vi "PE_DataAcquisition_Expire.vi"() -> ()   [LabVIEW 2016]
uses:
  SerialSupport/Serial - Settings.ctl
  SerialSupport/Serial - XON-XOFF Characters.ctl
  SerialSupport/Serial - ASCII Characters.ctl
  <vilib>/Instr/_visa.llb/VISA Configure Serial Port (Instr).vi
  database/database.lvlib
panel:
  out "当前指令 2":string
  in  "标记 2":dbl
  in  "TestId 2":string
  out "CtrlCmdMsg":string
  out "串口信息发送持久化":bool=TRUE
  out "串口信息发送":bool=TRUE
  out "UDP发送持久化":bool=TRUE
  out "TCP发送持久化":bool=TRUE
  out "串口接收持久化":bool=TRUE
  in  "串口发送按钮":bool
  in  "Serial output":string caption="字符串输出"
  in  "终止符":u8=10 format="%.0x"
  in  "终止符时结束写入？":bool=TRUE
  in  "VISA资源名称":refnum<visa-resource-name>="COM10"
  in  "XON/XOFF字符":T1={"XON"=enum."DC1", "XOFF"=enum."DC3"}
  in  "串口设置":T3={"波特率"=115200, "数据位"=8, "校验"=enum."None", "停止位"=10, "流控制"=0} {"流控制" items=["无"=0, "XON/XOFF"=1, "RTS/CTS"=2, "DTR/DSR"=4]; "停止位" items=["1.0"=10, "1.5"=15, "2.0"=20]; "数据位" min=5 max=8 step=1; "波特率" items=["75"=75, "110"=110, "134"=134, "150"=150, "300"=300, "600"=600, "1200"=1200, "1800"=1800, "2400"=2400, "4800"=4800, "7200"=7200, "9600"=9600, "14400"=14400, "19200"=19200, "28800"=28800, "38400"=38400, "56000"=56000, "57600"=57600, "115200"=115200, "128000"=128000, "230400"=230400]}
  in  "终止符时结束读取？":bool=TRUE
  in  "读取":bool=TRUE
  in  "串口停止":bool
  in  "串口发送命令":string="{\"cmd\":\"CT_ON\",\"id\":\"C_FR\",on:true}"
  out "串口信息":string
  in  "串口最大字节":u32=1000
  out "当前指令":string
  in  "错误输入 16":errorcluster caption="错误输入"
  in  "TestId":string
  in  "dataLabel":string
  in  "content":string
  in  "msgid":dbl
  # "用于说明数据来源等 如串口"
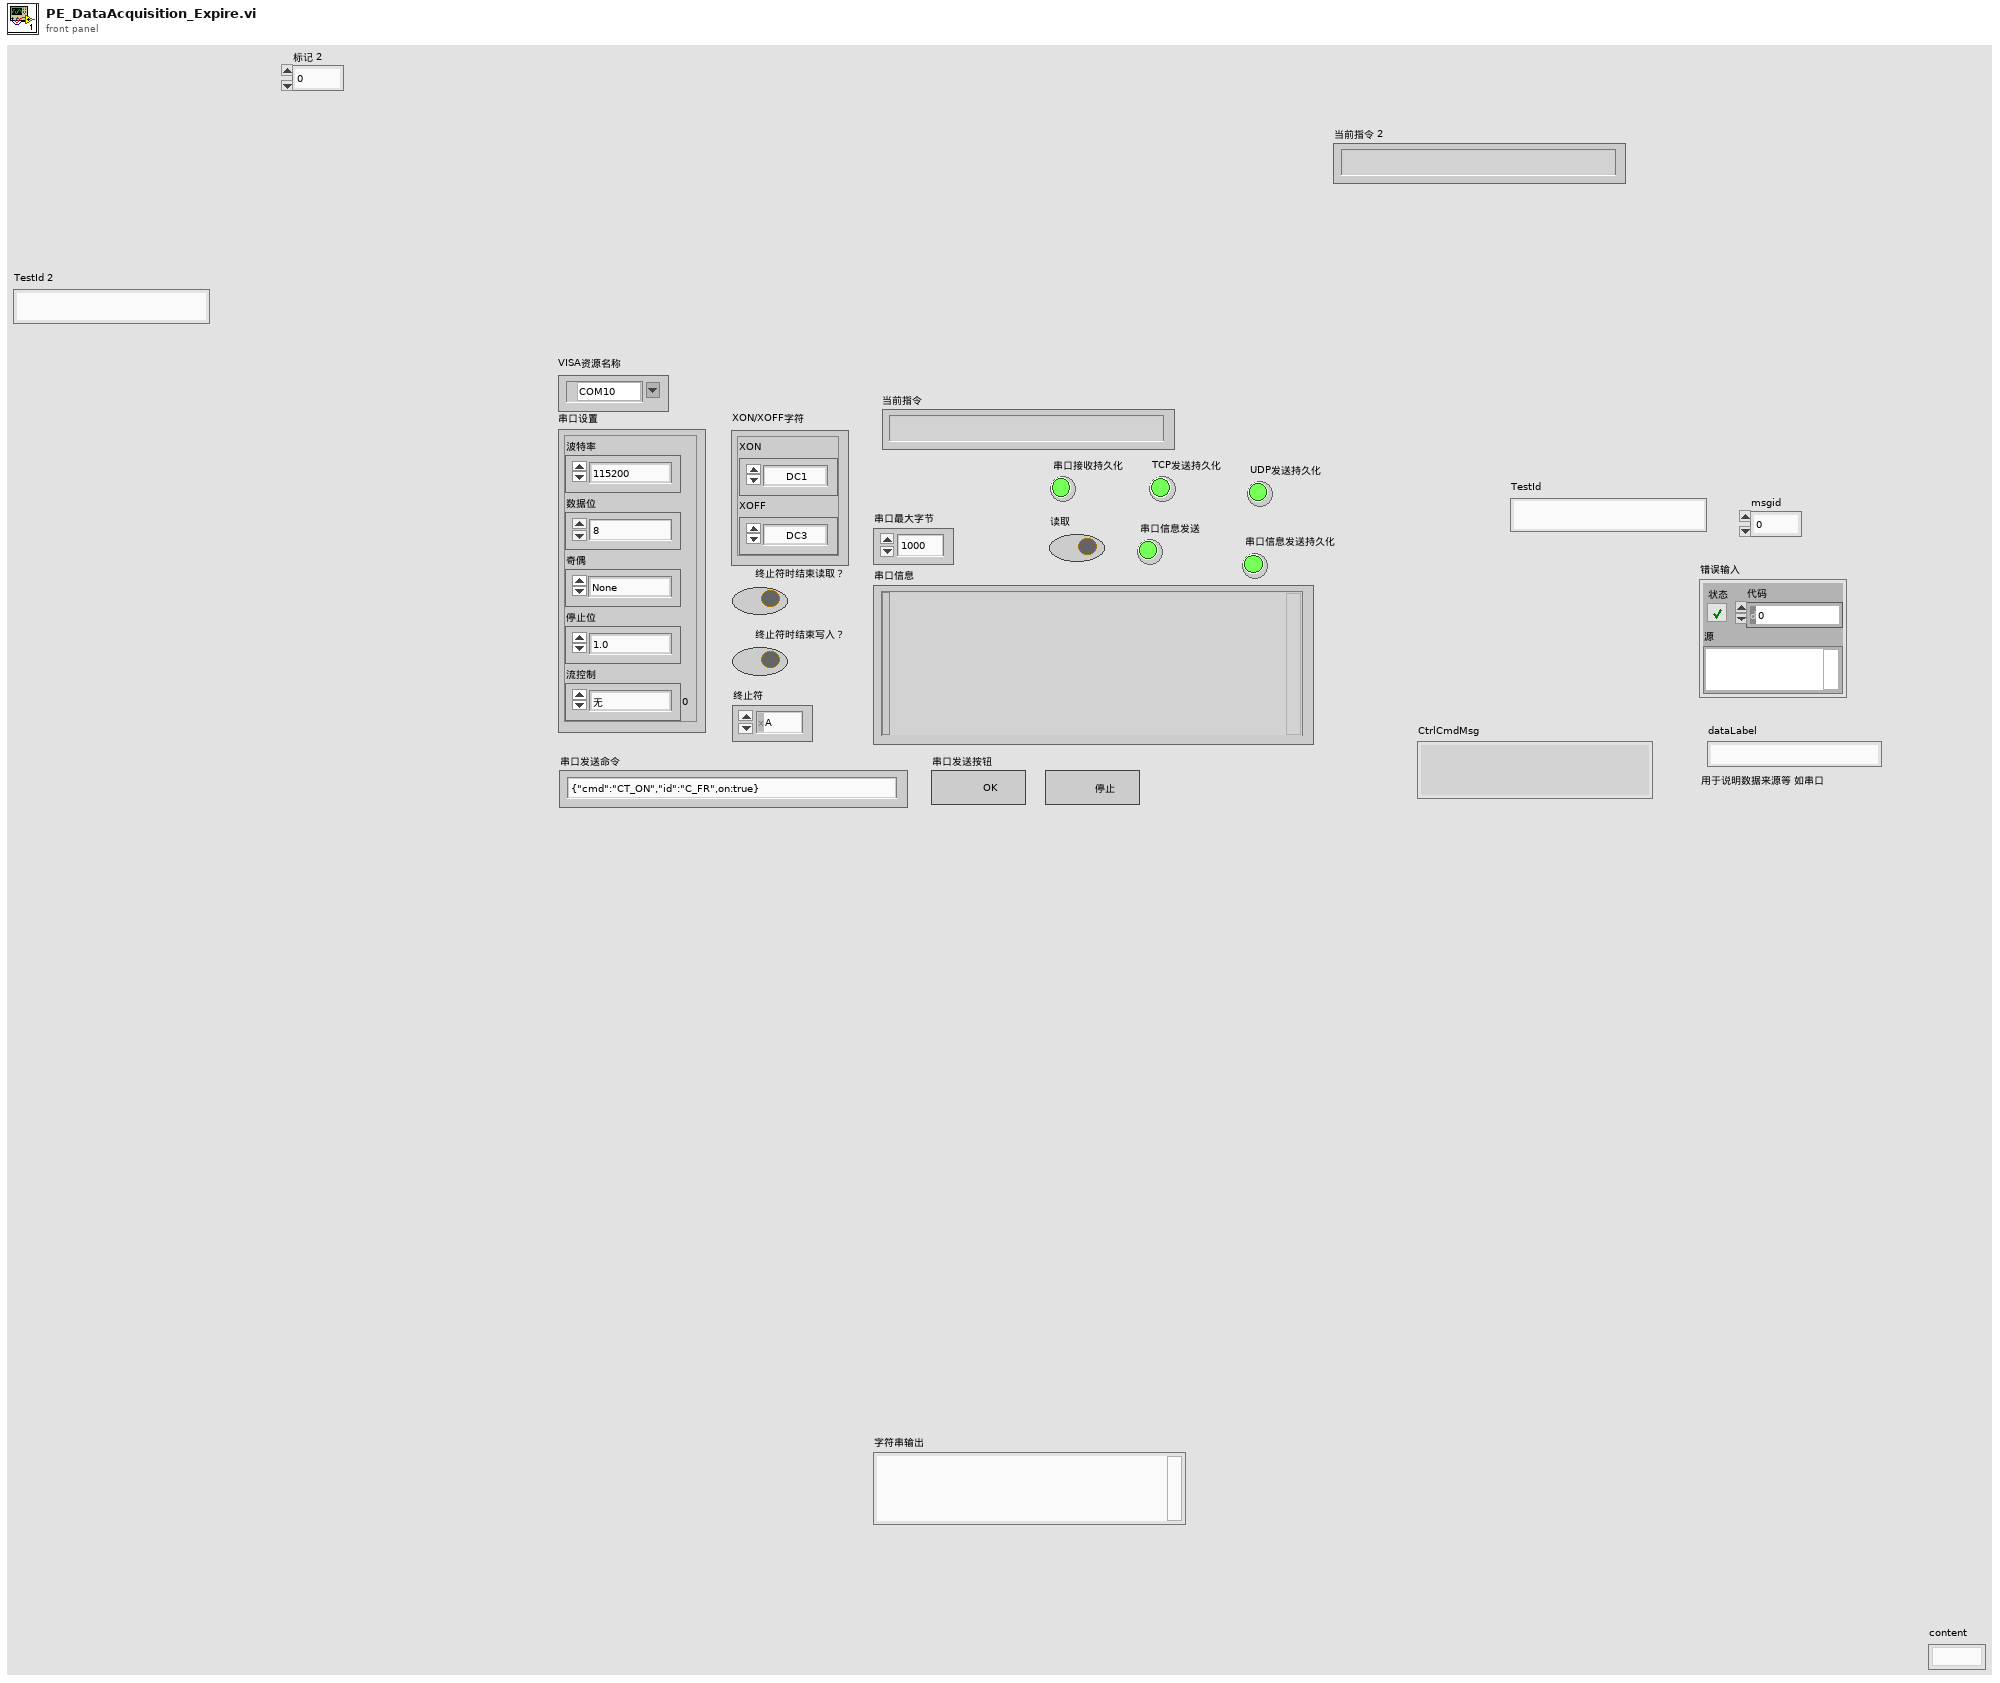
[diagram p1: front panel]
types:
  T1 = typedef "Serial - XON-XOFF Characters.ctl" = cluster{"XON":T2, "XOFF":T2}
  T2 = typedef "Serial - ASCII Characters.ctl" = enum16{"NUL", "SOH", "STX", "ETX", "EOT", "ENQ", "ACK", "BEL", "BS", "HT", "LF", "VT", "FF", "CR", "SO", "SI", "DLE", "DC1", "DC2", "DC3", "DC4", "NAK", "SYN", "ETB", "CAN", "EM", "SUB", "ESC", "FS", "GS", "RS", "US", "SP", "!", "\"", "#", "$", "%", "&", "'", "(", ")", "*", "+", ",", "- (-)", ".", "/", "0", "1", "2", "3", "4", "5", "6", "7", "8", "9", ":", ";", "<", "=", ">", "?", "@", "A", "B", "C", "D", "E", "F", "G", "H", "I", "J", "K", "L", "M", "N", "O", "P", "Q", "R", "S", "T", "U", "V", "W", "X", "Y", "Z", "[", "\\", "]", "^", "_", "`", "a", "b", "c", "d", "e", "f", "g", "h", "i", "j", "k", "l", "m", "n", "o", "p", "q", "r", "s", "t", "u", "v", "w", "x", "y", "z", "{", "|", "}", "~"}
  T3 = typedef "Serial - Settings.ctl" = cluster{"波特率":u32, "数据位":u16, "校验":enum16{"None", "Odd", "Even", "Mark", "Space"}, "停止位":u16, "流控制":u16}
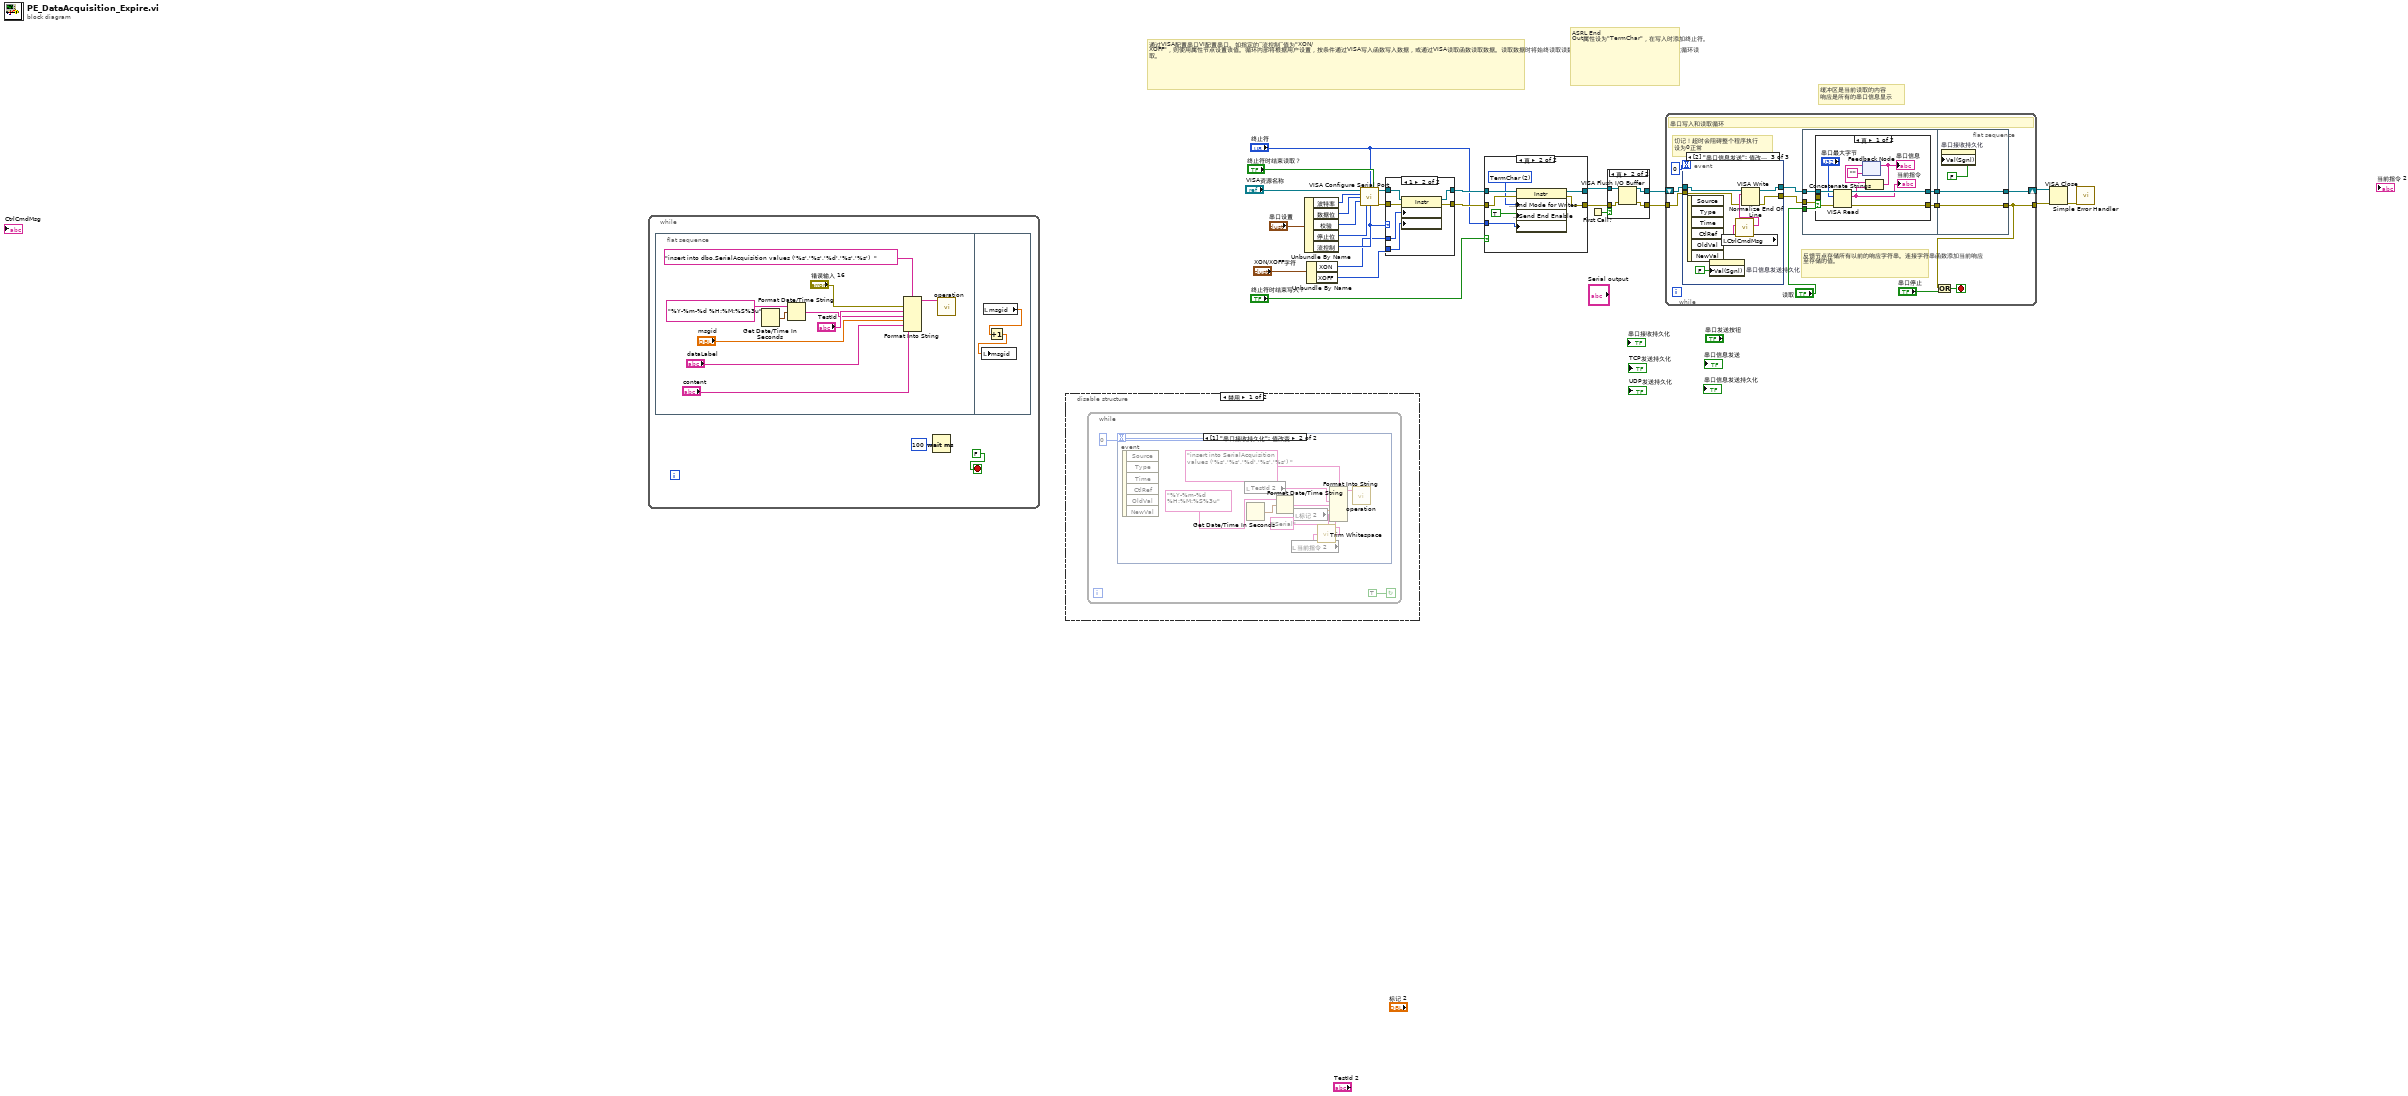
[diagram p0: block diagram]
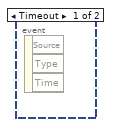
[diagram p2: hidden frame]
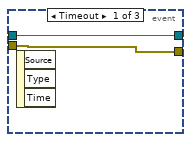
[diagram p8: hidden frame]
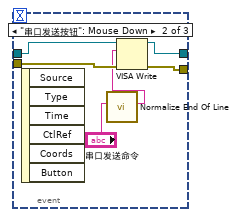
[diagram p9: hidden frame]
diagram:
  # "缓冲区是当前读取的内容\n响应是所有的串口信息显示"
  # "ASRL End Out属性设为\"TermChar\"，在写入时添加终止符。"
  # "通过VISA配置串口VI配置串口。如指定的“流控制”值为\"XON/XOFF\"，则使用属性节点设置该值。循环内部将根据用户设置，按条件通过VISA写入函数写入数据，或通过VISA读取函数读取数据。读取数据时将始终读取读数值指定的数据数量。多余数据将在下一次循环读取。"
  n1 = while {
    stop <- FALSE stop-if-true
    n2 = flat-sequence {
      frame #0 {
        n3 = Get Date/Time In Seconds() -> (seconds since 1Jan1904=w34:timestamp)
        n4 = Format Date/Time String ("格式化日期/时间字符串")(time format string (%c)="%Y-%m-%d %H:%M:%S%3u" ("时间格式字符串(%c)"), seconds (now)=w34) -> (date/time string=w29:string)  [unwired: 1 in]
        n5 = Format Into String(format string="insert into dbo.SerialAcquisition values ('%s','%s','%d','%s','%s')  " ("格式字符串"), error in="错误输入 16", "TestId", w29, "msgid", "dataLabel", "content") -> (resulting string=w37:string)  [unwired: 1 in, 1 out]
        n6 = call "operation.vi"("Command Text"=w37) -> ()  [unwired: 9 in, 1 out]
      }
      frame #1 {
        n7 = local read "msgid"() -> (w38:dbl)
        n8 = Increment(x=w38) -> (x+1=w39:dbl)
        n9 = local write "msgid"(w39) -> ()
      }
    }
    n10 = Wait (ms)(milliseconds to wait=u32 100) -> ()  [unwired: 1 out]
  }
  n11 = disable-structure shown="禁用" {
    frame Disabled {
      n12 = while {
        stop <- TRUE continue-if-true
        n13 = event shown="[1] \"串口接收持久化\": 值改变" {
          selector: _ -> [_ _]
          dyn-events: _ -> [_ _]
          timeout: 0 -> [_ _]
          event Timeout {
            n14 = event-data() -> ()  [unwired: 1 in, 3 out]
          }
          event "串口接收持久化": Value Change {
            n15 = event-data() -> ()  [unwired: 1 in, 6 out]
            n16 = local read "TestId 2"() -> (w47:string)
            n17 = Get Date/Time In Seconds() -> (seconds since 1Jan1904=w48:timestamp)
            n18 = Format Date/Time String ("格式化日期/时间字符串")(time format string (%c)="%Y-%m-%d %H:%M:%S%3u" ("时间格式字符串(%c)"), seconds (now)=w48) -> (date/time string=w49:string)  [unwired: 1 in]
            n19 = local read "当前指令 2"() -> (w44:string)
            n20 = local read "标记 2"() -> (w50:dbl)
            n21 = call <vilib>:"Trim Whitespace.vi"("string"=w44) -> ("trimmed string"=w43:string)  [unwired: 1 in]
            n22 = Format Into String(format string="insert into SerialAcquisition values ('%s','%s','%d','%s','%s') " ("格式字符串"), w47, w49, w50, "Serial" ("input 4"), w43) -> (resulting string=w46:string)  [unwired: 2 in, 1 out]
            n23 = call "operation.vi"("Command Text"=w46) -> ()  [unwired: 9 in, 1 out]
          }
        }
      }
    }
    frame Enabled {
    }
  }
  n24 = Unbundle By Name("串口设置") -> ("波特率"=w18:u32, "数据位"=w19:u16, "校验"=w20:enum16{"None", "Odd", "Even", "Mark", "Space"}, "停止位"=w21:u16, "流控制"=w12:u16)
  n25 = Unbundle By Name("XON/XOFF字符") -> ("XON"=w11:T2, "XOFF"=w10:T2)
  n26 = call-poly "VISA Configure Serial Port"("VISA resource name"="VISA资源名称", "termination char\n(0xA = '\\n' = LF)"="终止符", "Enable Termination\nChar (T)"="终止符时结束读取？", "baud rate (9600)"=w18, "data bits (8)"=w19, "parity (0:none)"=w20, "stop bits (10: 1 bit)"=w21, "flow control (0:none)"=w12) -> ("VISA resource name out"=w22:refnum<visa-resource-name>, "error out"=w23:errorcluster)  [unwired: 2 in, 4 out]
  n27 = case shown="1" w12 {
    tunnel: [w52 w59] -> w9
    tunnel: [w53 w58] -> w8
    tunnel: w23 -> [w52 w57]
    tunnel: w22 -> [w53 w56]
    tunnel: w11 -> [_ w55]
    tunnel: w10 -> [_ w54]
    frame Default {
    }
    frame 1 {
      n28 = property class="Instr"(reference=w56, error in=w57, "Serial Settings:Flow Control XON Character"=w55, "Serial Settings:Flow Control XOFF Character"=w54) -> (reference out=w58:refnum<visa-resource-name>, error out=w59:errorcluster)
    }
  }
  n29 = case shown="真" "终止符时结束写入？" {
    tunnel: w8 -> [w60 w68]
    tunnel: w9 -> [w61 w67]
    tunnel: [w60 w66] -> w5
    tunnel: [w61 w65] -> w4
    tunnel: "终止符" -> [_ w63]
    frame False {
    }
    frame True {
      w64 = u16 2 items=["None", "LastBit", "TermChar", "Break"] ("Serial Settings:Serial End Mode for Writes")
      n30 = property class="Instr"(reference=w68, error in=w67, "Serial Settings:End Mode for Writes"=w64, "Message Based Settings:Send End Enable"=TRUE, "Message Based Settings:Termination Character"=w63) -> (reference out=w66:refnum<visa-resource-name>, error out=w65:errorcluster)
    }
  }
  n31 = First Call?() -> (First Call?: T/F=w1:bool)
  n32 = case shown="真" w1 {
    tunnel: w5 -> [w70 w74]
    tunnel: w4 -> [w69 w73]
    tunnel: [w70 w72] -> w3
    tunnel: [w69 w71] -> w2
    frame False {
    }
    frame True {
      n33 = VISA Flush I/O Buffer(VISA resource name=w74, error in (no error)=w73) -> (VISA resource name out=w72:refnum<visa-resource-name>, error out=w71:errorcluster)  [unwired: 1 in]
    }
  }
  n34 = while {
    shift-right: [w86] -> w13
    shift-left: w3 -> [w79]
    tunnel: w2 -> [w81]
    tunnel: [w83] -> w14
    stop <- w84 stop-if-true
    # "反馈节点存储所有以前的响应字符串。连接字符串函数添加当前响应至存储的值。"
    # "切记！超时会阻碍整个程序执行\n设为0正常"
    # "串口写入和读取循环"
    n35 = event shown="[2] \"串口信息发送\": 值改变" {
      selector: _ -> [_ _ _]
      dyn-events: _ -> [_ _ _]
      timeout: 0 -> [_ _ _]
      tunnel: w81 -> [w106 w113 w116]
      tunnel: [w106 w112 w117] -> w80
      tunnel: w79 -> [w107 w111 w119]
      tunnel: [w107 w110 w118] -> w78
      event Timeout {
        n36 = event-data() -> ()  [unwired: 1 in, 3 out]
      }
      event "串口发送按钮": Mouse Down {
        n37 = event-data() -> ()  [unwired: 1 in, 6 out]
        n38 = call <vilib>:"Normalize End Of Line.vi"("string in"="串口发送命令") -> ("string out"=w108:string)  [unwired: 7 in]
        n39 = VISA Write(VISA resource name=w111, write buffer=w108, error in (no error)=w113) -> (VISA resource name out=w110:refnum<visa-resource-name>, error out=w112:errorcluster)  [unwired: 1 out]
      }
      event "串口信息发送": Value Change {
        n40 = event-data() -> ()  [unwired: 1 in, 6 out]
        n41 = property on="串口信息发送持久化" class="Bool (严格)"("Val(Sgnl)"=FALSE ("Value (Signaling)")) -> ()  [unwired: 2 in, 2 out]
        n42 = local read "CtrlCmdMsg"() -> (w115:string)
        n43 = call <vilib>:"Normalize End Of Line.vi"("string in"=w115) -> ("string out"=w120:string)  [unwired: 7 in]
        n44 = VISA Write(VISA resource name=w119, write buffer=w120, error in (no error)=w116) -> (VISA resource name out=w118:refnum<visa-resource-name>, error out=w117:errorcluster)  [unwired: 1 out]
      }
    }
    n45 = flat-sequence {
      tunnel: "读取" -> [w90]
      tunnel: w80 -> [w88]
      tunnel: w78 -> [w87]
      tunnel: [w91] -> w76
      tunnel: [w89] -> w75
      tunnel: [w104] -> w83
      tunnel: [w105] -> w86
      tunnel: w76 -> [w105]
      tunnel: w75 -> [w104]
      frame #0 {
        n46 = case shown="真" w90 {
          tunnel: [w98 w102] -> w91
          tunnel: w87 -> [w100 w102]
          tunnel: [w96 w101] -> w89
          tunnel: w88 -> [w99 w101]
          frame True {
            n47 = VISA Read(VISA resource name=w100, byte count="串口最大字节", error in (no error)=w99) -> (VISA resource name out=w98:refnum<visa-resource-name>, read buffer=w92:string, error out=w96:errorcluster)  [unwired: 1 out]
            "当前指令" <- w92
            n48 = feedback #1("") -> (w95:string)
            n49 = Concatenate Strings(w95, w92) -> (w94:string)
            "串口信息" <- w94
            n50 = feedback-in #1(w94) -> ()
          }
          frame False {
          }
        }
      }
      frame #1 {
        n51 = property on="串口接收持久化" class="Bool (严格)"("Val(Sgnl)"=FALSE ("Value (Signaling)")) -> ()  [unwired: 2 in, 2 out]
      }
    }
    n52 = Or(x=w83, y="串口停止") -> (x .or. y?=w84:bool)
  }
  n53 = VISA Close(VISA resource name=w13, error in (no error)=w14) -> (error out=w15:errorcluster)
  n54 = call <vilib>:"Simple Error Handler.vi"("error in (no error)"=w15) -> ()  [unwired: 1 in, 8 out]
